vi "Main.vi"(8 "error in":errorcluster, 11 "Alarm Worker in":refnum<class "Alarm Worker.lvclass">) -> (0 "error out":errorcluster, 3 "Alarm Worker out":refnum<class "Alarm Worker.lvclass">)   [LabVIEW 2020, in "Alarm Worker.lvclass"]
doc: "The <b>Queued Message Handler</b> of the Worker that owns this VI."
uses:
  Alarm Worker.lvclass
  C:/Program Files (x86)/National Instruments/LabVIEW 2020/vi.lib/addons/_Workers/Library/Classes/Worker/Worker.lvclass
  Initialization Data.ctl
  Response Cases.ctl
  Alarm Worker.lvclass/Alarm Worker.ctl
  Base Classes/BaseView/rqp_InsertPanel.ctl
  <vilib>/addons/_Workers/Library/Classes/Message Queue/Message Queue.lvclass
  Base Classes/BaseView/BaseView.lvclass
panel:
  out "Alarm":string
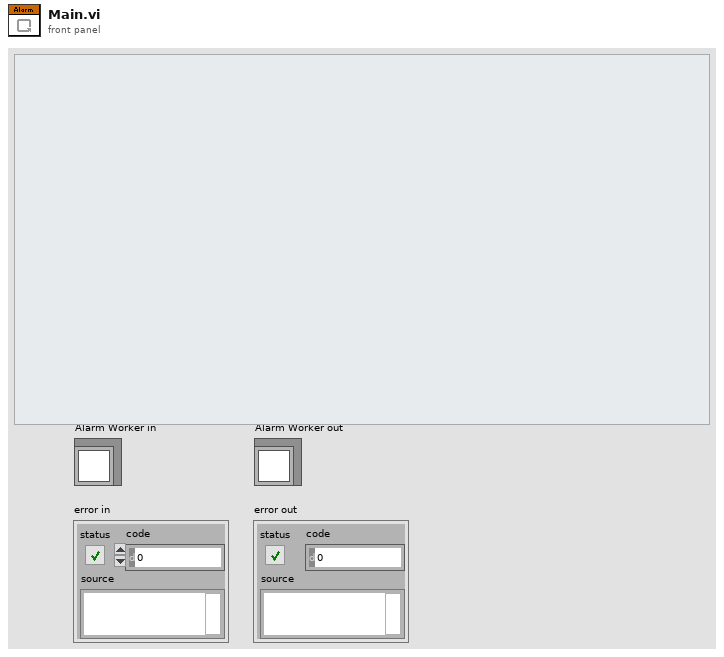
[diagram p1: front panel]
types:
  T1 = typedef "Alarm Worker.lvclass/Initialization Data.ctl" = cluster{"Response Cases":T2}
  T2 = typedef "Alarm Worker.lvclass/Response Cases.ctl" = cluster{"Placeholder - Can be deleted":string}
  T3 = typedef "BaseView.lvclass/rqp_InsertPanel.ctl" = cluster{"SubPanel":refnum<vi>}
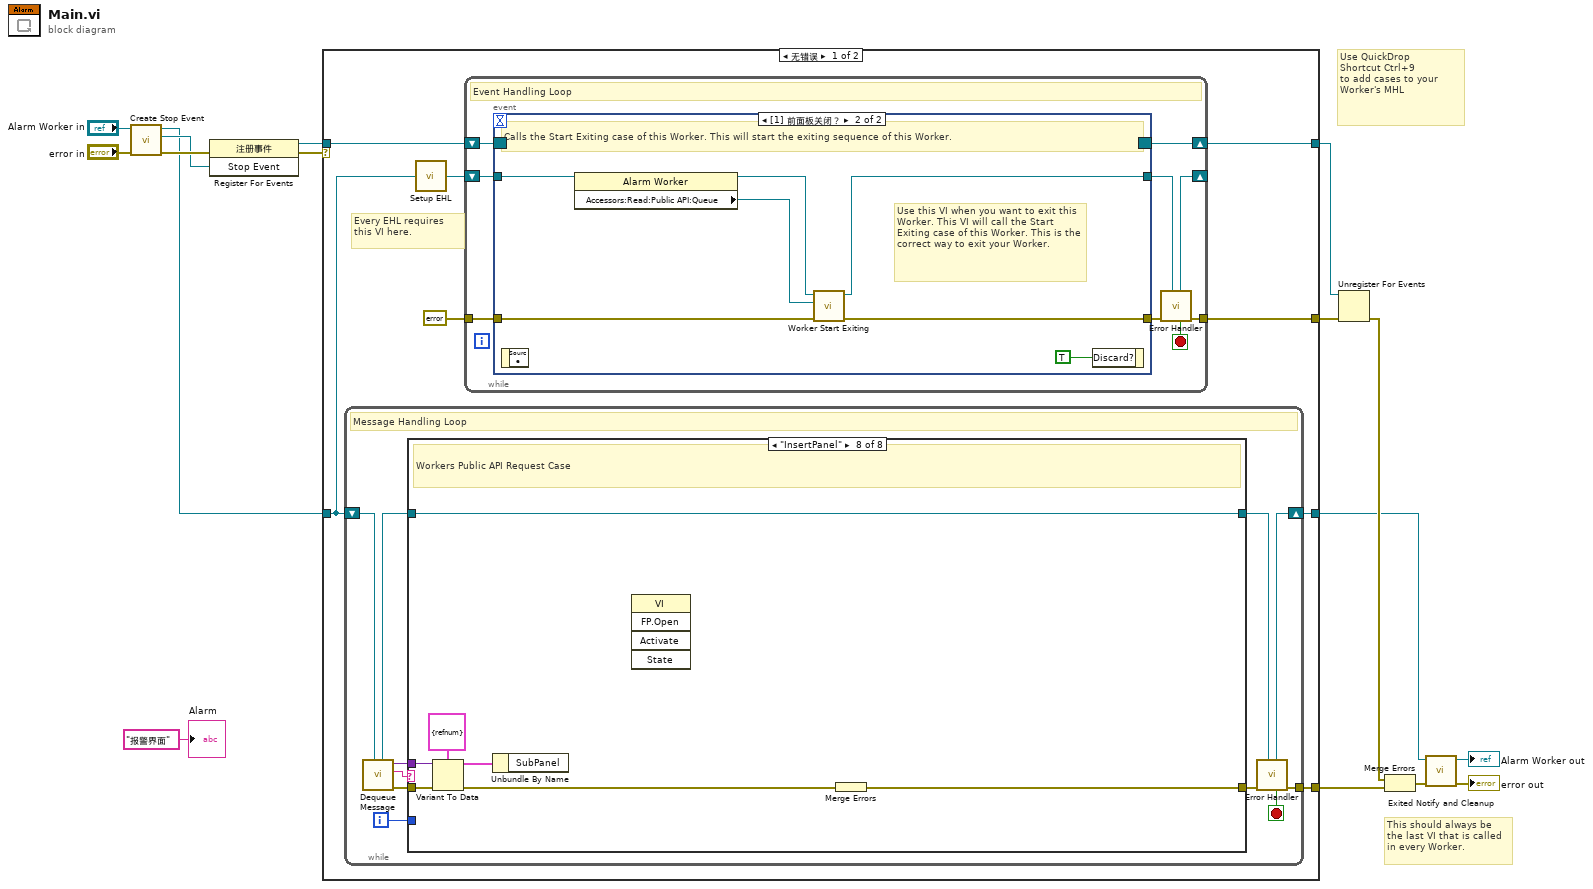
[diagram p0: block diagram]
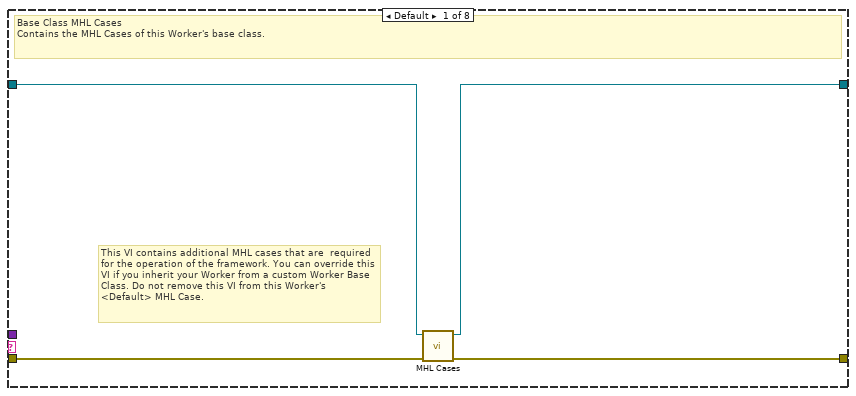
[diagram p2: hidden frame]
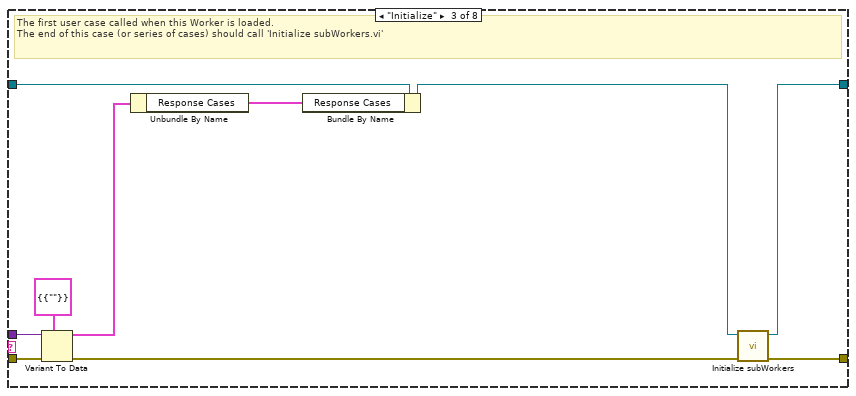
[diagram p4: hidden frame]
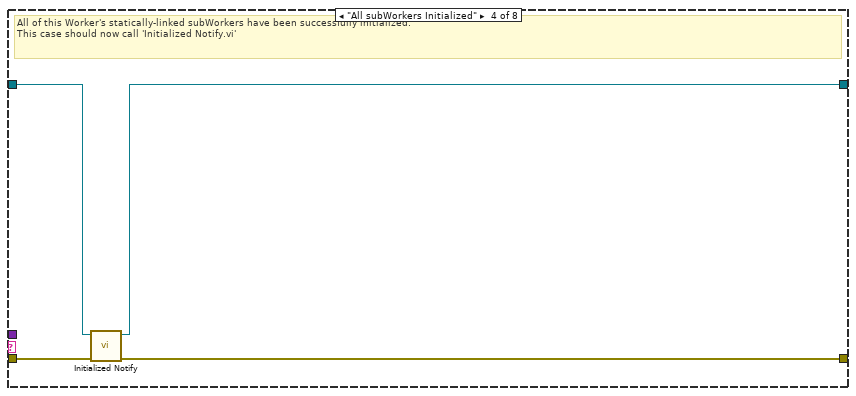
[diagram p5: hidden frame]
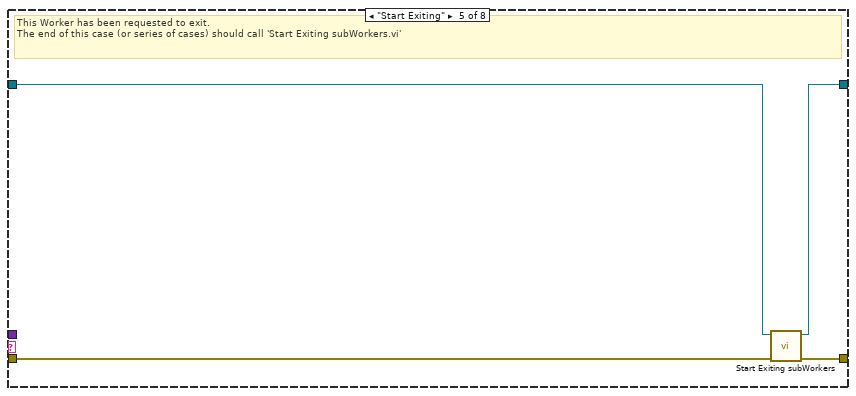
[diagram p6: hidden frame]
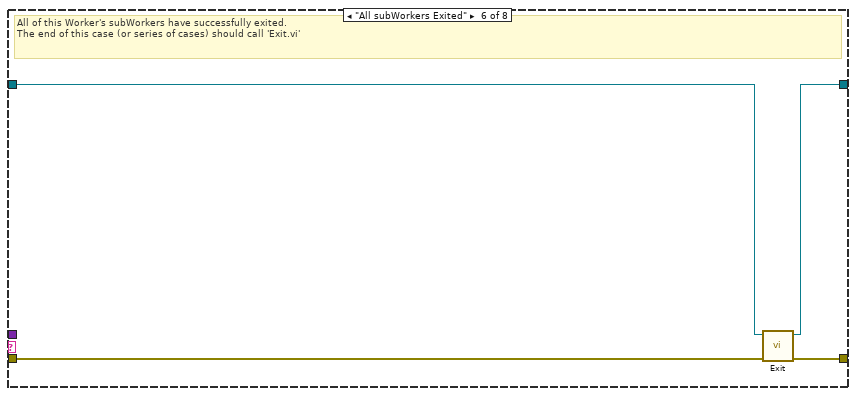
[diagram p7: hidden frame]
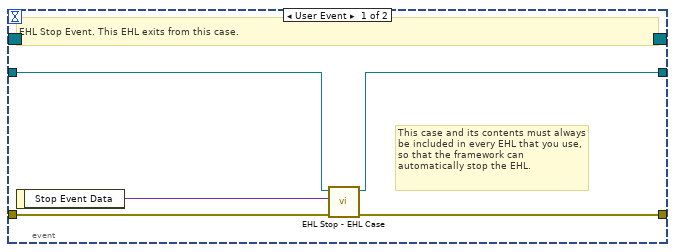
[diagram p9: hidden frame]
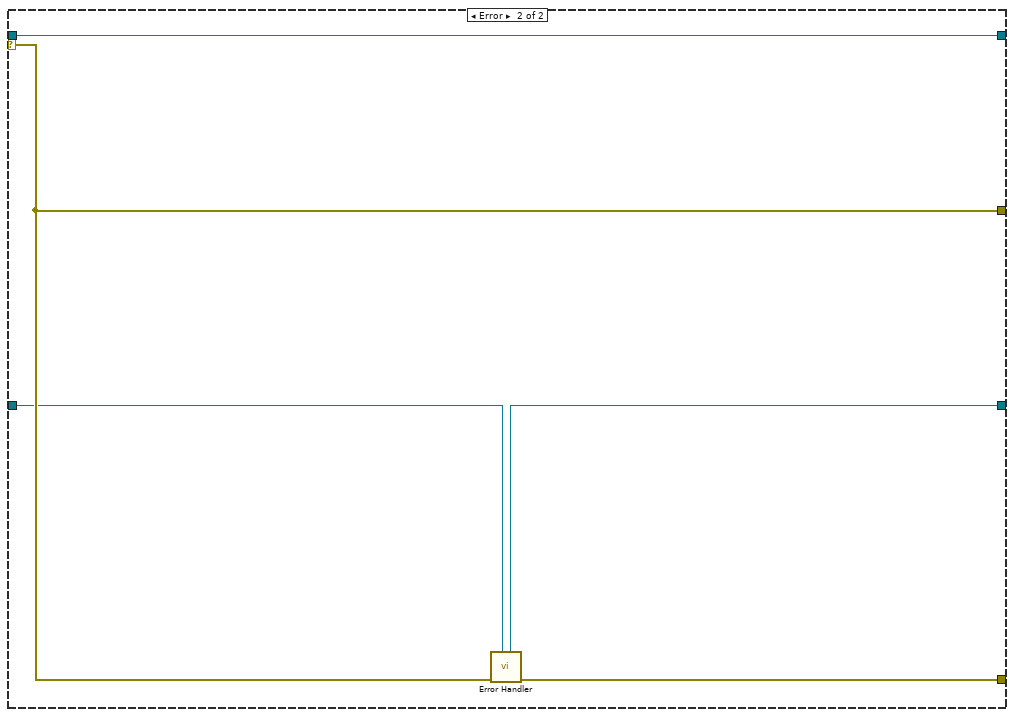
[diagram p10: hidden frame]
diagram:
  # "Use QuickDrop\nShortcut Ctrl+9\nto add cases to your\nWorker's MHL"
  # "This should always be the last VI that is called in every Worker."
  n1 = call-dynamic "Create Stop Event.vi"("error in"="error in", "Worker"="Alarm Worker in") -> ("error out"=w11:errorcluster, "Stop Event"=w8:refnum<user-event>, "Worker out"=w5:refnum<class "Alarm Worker.lvclass">)  [unwired: 7 in]
  n2 = register-events(error in=w11, w8) -> (reference out=w10:refnum<event-registration>, error out=w2:errorcluster)  [unwired: 1 in]
  n3 = case shown="无错误" w2 {
    tunnel: w5 -> [w19 w95]
    tunnel: [w17 w96] -> w9
    tunnel: w10 -> [w24 w97]
    tunnel: [w21 w98] -> w15
    tunnel: [w23 w97] -> w14
    tunnel: [w18 w94] -> w12
    selector: w2 -> [_ w98]
    frame No Error {
      # "Every EHL requires\nthis VI here."
      n4 = while {
        shift-right: [w33] -> w18
        shift-left: w19 -> [w35]
        tunnel: [w34] -> w17
        i -> [w26]
        stop <- w27 stop-if-true
        # "Message Handling Loop"
        n5 = call-dynamic "Dequeue Message.vi"("Worker"=w35) -> ("error out"=w32:errorcluster, "Case out"=w28:string, "Data out"=w25:variant, "Worker out"=w30:refnum<class "Alarm Worker.lvclass">)  [unwired: 6 in, 1 out]
        n6 = case "Worker MHL Case Structure (DO NOT CHANGE LABEL NAME)" shown="\"InsertPanel\"" w28 {
          tunnel: w32 -> [w39 w40 w49 w53 w56 w63 w65 w71]
          tunnel: [w38 w40 w51 w52 w59 w62 w65 w66] -> w31
          tunnel: w30 -> [w37 w41 w48 w55 w57 w61 w64 w72]
          tunnel: [w36 w41 w50 w54 w58 w60 w64 w72] -> w29
          tunnel: w26 -> [_ _ _ _ _ _ _ _]
          tunnel: w25 -> [_ _ w46 _ _ _ _ w68]
          frame Default {
            # "This VI contains additional MHL cases that are  required for the operation of the framework. You can override this VI if you inherit your Worker from a custom Worker Base Class. Do not remove this VI from this Worker's <Default> MHL Case."
            # "Base Class MHL Cases\nContains the MHL Cases of this Worker's base class."
            n7 = call-dynamic "MHL Cases.vi"("error in"=w39, "BaseView in"=w37) -> ("error out"=w38:errorcluster, "BaseView out"=w36:refnum<class "Alarm Worker.lvclass">)  [unwired: 8 in]
          }
          frame "------------ FRAMEWORK CASES -----------" {
            # "Start of Workers Framework Cases"
          }
          frame "Initialize" {
            # "The first user case called when this Worker is loaded.\nThe end of this case (or series of cases) should call 'Initialize subWorkers.vi'"
            n8 = Variant To Data(error in=w49, type=T1 {"Response Cases"={"Placeholder - Can be deleted"=""}} ("Initialization Data"), Variant=w46) -> (data=w44:T1, error out=w47:errorcluster)
            n9 = Unbundle By Name(w44) -> ("Response Cases"=w43:T2)
            n10 = Bundle By Name(cluster=w48, "Response Cases"=w43) -> (w45:refnum<class "Alarm Worker.lvclass">)
            n11 = call-dynamic "Initialize subWorkers.vi"("error in"=w47, "Worker"=w45) -> ("error out"=w51:errorcluster, "dup Worker out"=w50:refnum<class "Alarm Worker.lvclass">)  [unwired: 8 in]
          }
          frame "All subWorkers Initialized" {
            # "All of this Worker's statically-linked subWorkers have been successfully initialized.\nThis case should now call 'Initialized Notify.vi'"
            n12 = call-dynamic "Initialized Notify.vi"("error in"=w53, "Worker"=w55) -> ("error out"=w52:errorcluster, "dup Worker out"=w54:refnum<class "Alarm Worker.lvclass">)  [unwired: 8 in]
          }
          frame "Start Exiting" {
            # "This Worker has been requested to exit. \nThe end of this case (or series of cases) should call 'Start Exiting subWorkers.vi'"
            n13 = call-dynamic "Start Exiting subWorkers.vi"("error_in"=w56, "Worker"=w57) -> ("error out"=w59:errorcluster, "dup Worker out"=w58:refnum<class "Alarm Worker.lvclass">)  [unwired: 8 in]
          }
          frame "All subWorkers Exited" {
            # "All of this Worker's subWorkers have successfully exited. \nThe end of this case (or series of cases) should call 'Exit.vi'"
            n14 = call-dynamic "Exit.vi"("error_in"=w63, "Worker"=w61) -> ("error out"=w62:errorcluster, "dup Worker out"=w60:refnum<class "Alarm Worker.lvclass">)  [unwired: 8 in]
          }
          frame "------------- PUBLIC API CASES -------------" {
            # "Start of Workers Public API Cases"
          }
          frame "InsertPanel" {
            # "Workers Public API Request Case"
            n15 = Variant To Data(error in=w71, type=T3 {"SubPanel"=refnum} ("Data"), Variant=w68) -> (data=w67:T3, error out=w70:errorcluster)
            n16 = Unbundle By Name(w67) -> ()  [unwired: 1 out]
            n17 = invoke class="VI" method="FP.Open"() -> ()  [unwired: 5 in, 5 out]
            n18 = Merge Errors(w70) -> (w66:errorcluster)
          }
        }
        n19 = call-dynamic "Error Handler.vi"("Worker"=w29, "error_in"=w31) -> ("error out"=w34:errorcluster, "Stop Loop"=w27:bool, "Worker out"=w33:refnum<class "Alarm Worker.lvclass">)  [unwired: 7 in]
      }
      n20 = call-dynamic "Setup EHL.vi"("Worker"=w19) -> ("Worker out"=w20:refnum<class "Alarm Worker.lvclass">)  [unwired: 14 in]
      n21 = while "Event Handling Loop" {
        shift-right: [w81] -> w23
        shift-left: w24 -> [w80]
        tunnel: [w76] -> w21
        tunnel: errorcluster {"status"=FALSE, "code"=0, "source"=""} ("error constant") -> [w78]
        shift-right: [w74] -> _
        shift-left: w20 -> [w79]
        stop <- w73 stop-if-true
        # "Event Handling Loop"
        n22 = event shown="[1] 前面板关闭？" {
          selector: w80 -> [_ _]
          dyn-events: [_ _] -> w81
          timeout: _ -> [_ _]
          tunnel: [w85 w92] -> w77
          tunnel: w78 -> [w86 w91]
          tunnel: w79 -> [w84 w90]
          tunnel: [w83 w89] -> w75
          event User Event {
            # "This case and its contents must always be included in every EHL that you use, so that the framework can automatically stop the EHL."
            # "EHL Stop Event. This EHL exits from this case."
            n23 = event-data() -> ("Stop Event Data"=w82:variant)  [unwired: 1 in]
            n24 = call-dynamic "EHL Stop - EHL Case.vi"("error in"=w86, "Stop Event Data"=w82, "Worker"=w84) -> ("error out"=w85:errorcluster, "Worker out"=w83:refnum<class "Alarm Worker.lvclass">)  [unwired: 7 in]
          }
          event Panel Close? {
            # "Use this VI when you want to exit this Worker. This VI will call the Start Exiting case of this Worker. This is the correct way to exit your Worker."
            # "Calls the Start Exiting case of this Worker. This will start the exiting sequence of this Worker."
            n25 = event-data() -> ()  [unwired: 1 in, 1 out]
            n26 = property class="Alarm Worker"(reference=w90) -> (reference out=w88:refnum<class "Alarm Worker.lvclass">, "Accessors:Read:Public API:Queue"=w87:refnum<class "Message Queue.lvclass">)  [unwired: 1 in, 1 out]
            n27 = call-dynamic "Worker Start Exiting.vi"("error_in"=w91, "Message Queue"=w87, "Worker"=w88) -> ("error out"=w92:errorcluster, "dup Worker out"=w89:refnum<class "Alarm Worker.lvclass">)  [unwired: 7 in]
            n28 = event-data("Discard?"=TRUE) -> ()  [unwired: 1 in, 1 out]
          }
        }
        n29 = call-dynamic "Error Handler.vi"("Worker"=w75, "error_in"=w77) -> ("error out"=w76:errorcluster, "Stop Loop"=w73:bool, "Worker out"=w74:refnum<class "Alarm Worker.lvclass">)  [unwired: 7 in]
      }
    }
    frame Error {
      n30 = call-dynamic "Error Handler.vi"("Worker"=w95, "error_in"=w98) -> ("error out"=w96:errorcluster, "Worker out"=w94:refnum<class "Alarm Worker.lvclass">)  [unwired: 7 in, 1 out]
    }
  }
  n31 = Unregister For Events(event registration refnum=w14, error in=w15) -> (error out=w16:errorcluster)
  n32 = Merge Errors(w16, w9) -> (w13:errorcluster)
  n33 = call-dynamic "Exited Notify and Cleanup.vi"("error_in"=w13, "Worker"=w12) -> ("error out"=→"error out":errorcluster, "dup Worker out"=→"Alarm Worker out":refnum<class "Alarm Worker.lvclass">)  [unwired: 8 in]
  "Alarm" <- "报警界面" ("Alarm")
